vi "50019base64_fast_decode.vi"(8 "error in (no error)":errorcluster, 10 "string in (base64-encoded)":string) -> (0 "error out":errorcluster, 2 "string out (decoded)":string)   [LabVIEW 8.6]
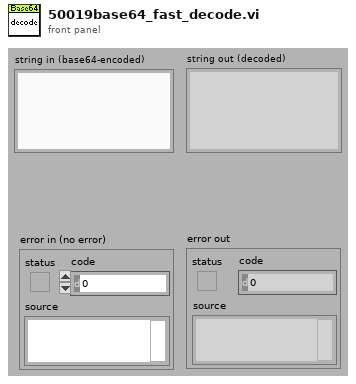
[diagram p1: front panel]
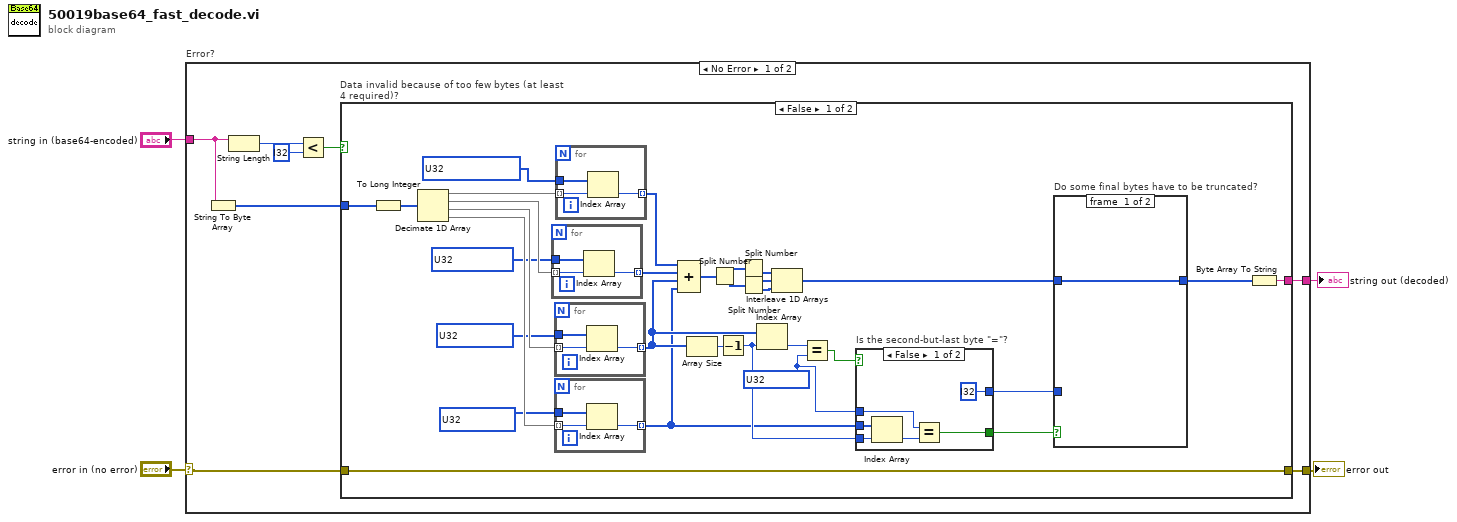
[diagram p0: block diagram]
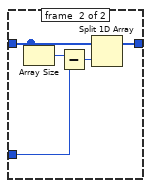
[diagram p2: hidden frame]
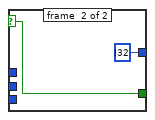
[diagram p3: hidden frame]
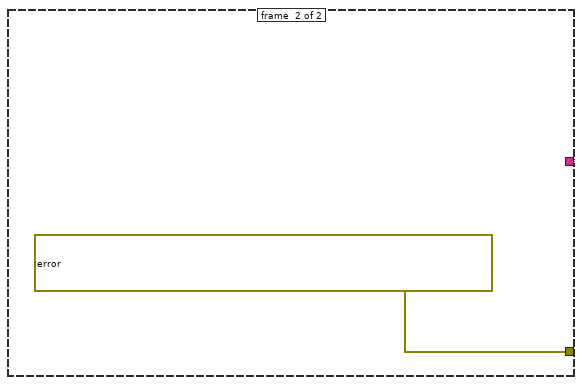
[diagram p4: hidden frame]
diagram:
  n1 = case "Error?" shown="No Error" "error in (no error)" {
    selector: "error in (no error)" -> [w7 w72]
    tunnel: "string in (base64-encoded)" -> [w11 _]
    tunnel: [w6 w72] -> w3
    tunnel: [w5 _] -> w1
    frame #0 {
      n2 = String To Byte Array(string=w11) -> (unsigned byte array=w10:u8[])
      n3 = String Length(string=w11) -> (length=w8:i32)
      n4 = Less?(x=w8, y=i32 ?) -> (x < y?=w9:bool)
      n5 = case "Data invalid because of too few bytes (at least 4 required)?" shown="False" w9 {
        tunnel: w10 -> [w25 _]
        tunnel: [w43 string ?] -> w5
        tunnel: [w13 errorcluster ? ("error IO")] -> w6
        tunnel: w7 -> [w13 _]
        frame #0 {
          w18 = u32 ? ("y")
          n6 = To Long Integer(number=w25) -> (32bit integer=w42:i32[])
          n7 = Decimate 1D Array(w42) -> (w31:i32[], w41:i32[], w32:i32[], w30:i32[])
          n8 = for {
            tunnel: w41 -> [w65] mode=indexing
            tunnel: u32[] ? ("array 3") -> [w66]
            tunnel: [w64] -> w39 mode=indexing
            n9 = Index Array(array=w66, index=w65) -> (element=w64:u32)
          }
          n10 = for {
            tunnel: u32[] ? ("array 2") -> [w63]
            tunnel: [w62] -> w23 mode=indexing
            tunnel: w32 -> [w61] mode=indexing
            n11 = Index Array(array=w63, index=w61) -> (element=w62:u32)
          }
          n12 = for {
            tunnel: u32[] ? ("Array") -> [w60]
            tunnel: [w59] -> w21 mode=indexing
            tunnel: w30 -> [w58] mode=indexing
            n13 = Index Array(array=w60, index=w58) -> (element=w59:u32)
          }
          n14 = for {
            tunnel: w31 -> [w68] mode=indexing
            tunnel: u32[] ? ("array 4") -> [w69]
            tunnel: [w67] -> w40 mode=indexing
            n15 = Index Array(array=w69, index=w68) -> (element=w67:u32)
          }
          n16 = Compound Arithmetic op=ADD(w40, w39, w23, w21) -> (w37:u32[])
          n17 = Array Size(array=w23) -> (size(s)=w24:i32)
          n18 = Split Number(x=w37) -> (hi(x)=w38:u16[], lo(x)=w36:u16[])
          n19 = Decrement(x=w24) -> (x-1=w22:i32)
          n20 = Split Number(x=w38) -> (lo(x)=w33:u8[])  [unwired: 1 out]
          n21 = Split Number(x=w36) -> (hi(x)=w34:u8[], lo(x)=w35:u8[])
          n22 = Index Array(array=w23, index=w22) -> (element=w20:u32)
          n23 = Interleave 1D Arrays(w33, w34, w35) -> (w15:u8[])
          n24 = Equal?(x=w20, y=w18) -> (x = y?=w19:bool)
          n25 = case "Is the second-but-last byte \"=\"?" shown="False" w19 {
            selector: w19 -> [_ w56]
            tunnel: w22 -> [w55 _]
            tunnel: w21 -> [w54 _]
            tunnel: w18 -> [w52 _]
            tunnel: [w51 w56] -> w17
            tunnel: [i32 ? i32 ?] -> w16
            frame #0 {
              n26 = Index Array(array=w54, index=w55) -> (element=w53:u32)
              n27 = Equal?(x=w52, y=w53) -> (x = y?=w51:bool)
            }
            frame #1 {
            }
          }
          n28 = case "Do some final bytes have to be truncated?" shown="True" w17 {
            tunnel: w16 -> [_ w49]
            tunnel: w15 -> [w44 w45]
            tunnel: [w44 w47] -> w14
            frame #0 {
            }
            frame #1 {
              n29 = Array Size(array=w45) -> (size(s)=w46:i32)
              n30 = Subtract(x=w46, y=w49) -> (x-y=w48:i32)
              n31 = Split 1D Array(array=w45, index=w48) -> (first subarray=w47:u8[])  [unwired: 1 out]
            }
          }
          n32 = Byte Array To String(unsigned byte array=w14) -> (string=w43:string)
        }
        frame #1 {
        }
      }
    }
    frame #1 {
    }
  }
  "error out" <- w3
  "string out (decoded)" <- w1
